vi "FTW-SQLite-Transaction-Begin.vi"(0 "SQLite Connector":refnum<class "FTW-SQLite-Connector.lvclass">, 11 "error in":errorcluster) -> (4 "SQLite Connector out":refnum<class "FTW-SQLite-Connector.lvclass">, 6 "Time to Execute+Compile":dbl format="%.6fsec", 8 "Time to Compile SQL":dbl format="%.6fsec", 15 "error out":errorcluster)   [LabVIEW 2015, in "FTW-SQLite-Connector.lvclass"]
uses:
  FTW-SQLite-Connector.lvclass
panel:
  # "Inputs"
  # "Outputs"
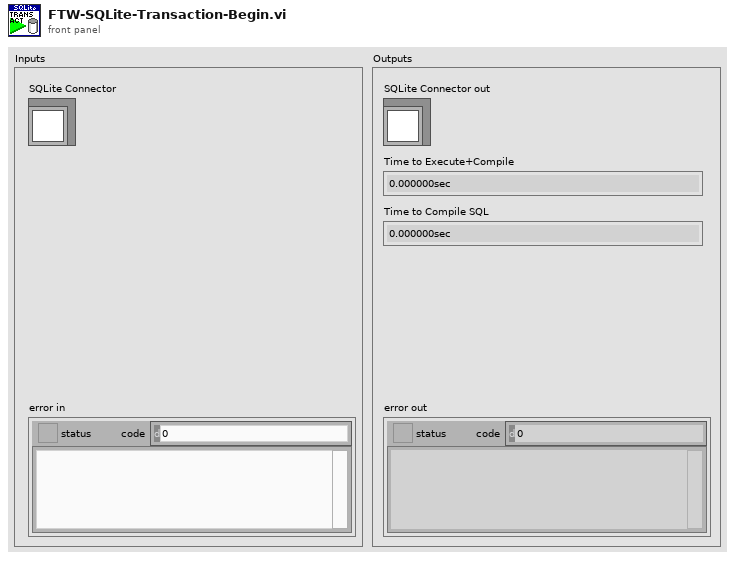
[diagram p1: front panel]
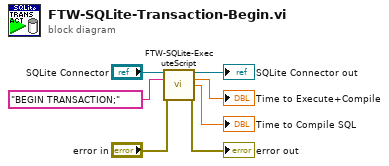
[diagram p0: block diagram]
diagram:
  n1 = call "FTW-SQLite-ExecuteScript.vi"("SQLite Connector"="SQLite Connector", "SQL Script"="BEGIN TRANSACTION;", "error in"="error in") -> ("SQLite Connector out"=→"SQLite Connector out":refnum<class "FTW-SQLite-Connector.lvclass">, "Time to Execute+Compile"=→"Time to Execute+Compile":dbl, "Time to Compile SQL"=→"Time to Compile SQL":dbl, "error out"=→"error out":errorcluster)  [unwired: 9 in]
